vi "Initial.vi"() -> (1 "flag":i32[](array[numeric]), 2 "Output cluster":T1)   [LabVIEW 2016]
uses:
  Model Management/Global_MdlMgmt.vi
  Communication/Global communication.vi
  <vilib>/imath/engines/lvmath2/RunTimeEngine/Managers/WorkSpace/UID Generator.vi
  <vilib>/imath/engines/lvmath2/RunTimeEngine/BuiltInFunctions/size/NIMS_[I32,I32]=size(GM).vi
  <vilib>/imath/engines/lvmath2/RunTimeEngine/RangeToken/NIMS_Range_R2 - Integer.vi
  <vilib>/imath/engines/lvmath2/RunTimeEngine/IndexRead/NIMS M(S,S).vi
  <vilib>/imathl/engines/lvmath/Functions/Error Handling/Create Error.vi
  <vilib>/imath/engines/lvmath2/RunTimeEngine/CommandStatement/MC_CommandStatement_break.vi
  <vilib>/imath/engines/lvmath2/RunTimeEngine/IndexRead/NIMS M($,S).vi
  <vilib>/imath/engines/lvmath2/RunTimeEngine/BuiltInFunctions/findnz/NIMS_[3o]_findnz(GColV).vi
  <vilib>/imath/engines/lvmath2/RunTimeEngine/ErrorHandling/NIMS_Create Error From Enums.vi
  <vilib>/imath/engines/lvmath2/RunTimeEngine/BuiltInFunctions/is_empty/NIMS_is_empty(GV).vi
  <vilib>/imath/engines/lvmath2/RunTimeEngine/BuiltInFunctions/size/NIMS_[I32,I32]=size(GCol).vi
  <vilib>/imath/engines/lvmath2/RunTimeEngine/IndexRead/NIMS V(S).vi
  <vilib>/imath/engines/lvmath2/RunTimeEngine/IndexRead/NIMS M(R2,$).vi
  <vilib>/imath/engines/lvmath2/RunTimeEngine/LocalVariableDefStatement/MC_LocalVariableDefStatement_Display.vi
  <vilib>/imath/engines/lvmath2/RunTimeEngine/RunTimeType/NIMS_RunTimeType_From StrictType (excl LVString).vi
  <vilib>/imath/engines/lvmath2/RunTimeEngine/IndexReplace/NIMS M(S,S)=S.vi
  <vilib>/imath/engines/lvmath2/RunTimeEngine/IndexRead/NIMS M(S,$).vi
  <vilib>/imath/engines/lvmath2/RunTimeEngine/MatrixToken/NIMS_MatrixToken_M_RV.vi
  <vilib>/imath/engines/lvmath2/RunTimeEngine/BuiltInFunctions/zeros/NIMS_V=zeros(I32,I32).vi
  <vilib>/imath/engines/lvmath2/RunTimeSupport/NIMS_Error if Not Equal.vi
  <vilib>/imath/engines/lvmath2/RunTimeEngine/IndexReplace/NIMS V(S)=S.vi
  <vilib>/imath/engines/lvmath2/RunTimeEngine/Managers/SymbolTable/Clear UID.vi
  <vilib>/imath/engines/lvmath2/RunTimeEngine/Managers/SymbolTable/NIMS_WorkSpace.lvlib
  <vilib>/imath/engines/lvmath2/RunTimeEngine/NodeEndStatement/NIMS_NodeEndStatement_Output.vi
  <vilib>/imath/engines/lvmath2/RunTimeEngine/ErrorHandling/NIMS_Finalize Error.vi
panel:
  in  "Tnumber":dbl=8.0
  out "PVmax":dbl
  out "fixedQ":dbl
  out "fixedP":dbl
  in  "PVramp":dbl=1000.0
  in  "maxV":dbl=1.05
  in  "minV":dbl=0.95
  in  "minf":dbl=59.5
  in  "maxf":dbl=60.5
  in  "Array 2":dbl[][](array[numeric])=[[1.0, 2.0, 3.0, 0.0, 100.0, 0.0, 0.0, 0.0, 0.0, 0.0, 0.0, 0.0, 0.0, 0.0, 0.0, 0.0], [2.0, 3.0, 1.0, 0.0, 1.0, 0.0, 0.0, 0.0, 0.0, 0.0, 0.0, 0.0, 0.0, 0.0, 0.0, 0.0], [3.0, 4.0, 1.0, 1.0, 2.0, 0.0, 0.0, 0.0, 0.0, 0.0, 0.0, 0.0, 0.0, 0.0, 0.0, 0.0], [4.0, 5.0, 1.0, 0.0, 4.0, 0.0, 0.0, 0.0, 0.0, 0.0, 0.0, 0.0, 0.0, 0.0, 0.0, 0.0], [4.0, 6.0, 3.0, 0.0, 100.0, 0.0, 0.0, 0.0, 0.0, 0.0, 0.0, 1.0, 2.0, 3.0, 0.0, 100.0], [3.0, 7.0, 1.0, 0.0, 3.0, 0.0, 0.0, 0.0, 0.0, 0.0, 0.0, 2.0, 3.0, 1.0, 0.0, 1.0], [7.0, 8.0, 1.0, 0.0, 5.0, 0.0, 0.0, 0.0, 0.0, 0.0, 0.0, 3.0, 4.0, 1.0, 0.0, 2.0], [7.0, 9.0, 1.0, 0.0, 6.0, 0.0, 0.0, 0.0, 0.0, 0.0, 0.0, 4.0, 5.0, 1.0, 0.0, 4.0], [9.0, 10.0, 1.0, 0.0, 7.0, 0.0, 0.0, 0.0, 0.0, 0.0, 0.0, 4.0, 6.0, 3.0, 0.0, 100.0], [10.0, 13.0, 2.0, 0.0, 100.0, 0.0, 0.0, 0.0, 0.0, 0.0, 0.0, 3.0, 7.0, 1.0, 0.0, 3.0], [10.0, 12.0, 2.0, 0.0, 100.0, 0.0, 0.0, 0.0, 0.0, 0.0, 0.0, 7.0, 8.0, 1.0, 0.0, 5.0], [10.0, 11.0, 1.0, 0.0, 8.0, 0.0, 0.0, 0.0, 0.0, 0.0, 0.0, 7.0, 9.0, 1.0, 0.0, 6.0], [11.0, 14.0, 3.0, 0.0, 100.0, 0.0, 0.0, 0.0, 0.0, 0.0, 0.0, 9.0, 10.0, 1.0, 0.0, 7.0], [0.0, 0.0, 0.0, 0.0, 0.0, 0.0, 0.0, 0.0, 0.0, 0.0, 0.0, 10.0, 13.0, 2.0, 0.0, 100.0], [0.0, 0.0, 0.0, 0.0, 0.0, 0.0, 0.0, 0.0, 0.0, 0.0, 0.0, 10.0, 12.0, 2.0, 0.0, 100.0], [0.0, 0.0, 0.0, 0.0, 0.0, 0.0, 0.0, 0.0, 0.0, 0.0, 0.0, 10.0, 11.0, 1.0, 0.0, 8.0], [0.0, 0.0, 0.0, 0.0, 0.0, 0.0, 0.0, 0.0, 0.0, 0.0, 0.0, 11.0, 14.0, 3.0, 0.0, 100.0]]
  out "error out":errorcluster
  in  "Array":dbl[][](array[numeric])=[[1.0, 0.0, 1.0, 0.0, 0.0, 0.0, 0.0, 0.0, 0.0, 0.0, 0.0, 0.0, 0.0, 0.0, 0.0, 0.0], [0.0, 0.0, 0.0, 0.0, 0.0, 0.0, 0.0, 0.0, 0.0, 0.0, 0.0, 0.0, 0.0, 0.0, 0.0, 0.0], [0.0, 0.0, 1.0, 1.0, 0.0, 0.0, 0.0, 0.0, 0.0, 0.0, 0.0, 0.0, 0.0, 0.0, 0.0, 0.0], [0.0, 0.0, 0.0, 0.0, 0.0, 0.0, 0.0, 0.0, 0.0, 0.0, 0.0, 0.0, 0.0, 0.0, 0.0, 0.0], [0.0, 0.0, 0.0, 0.0, 0.0, 0.0, 0.0, 0.0, 0.0, 0.0, 0.0, 1.0, 2.0, 3.0, 0.0, 100.0], [0.0, 0.0, 0.0, 0.0, 0.0, 0.0, 0.0, 0.0, 0.0, 0.0, 0.0, 2.0, 3.0, 1.0, 0.0, 1.0], [0.0, 0.0, 0.0, 0.0, 0.0, 0.0, 0.0, 0.0, 0.0, 0.0, 0.0, 3.0, 4.0, 1.0, 0.0, 2.0], [0.0, 0.0, 0.0, 0.0, 0.0, 0.0, 0.0, 0.0, 0.0, 0.0, 0.0, 4.0, 5.0, 1.0, 0.0, 4.0], [0.0, 0.0, 0.0, 0.0, 0.0, 0.0, 0.0, 0.0, 0.0, 0.0, 0.0, 4.0, 6.0, 3.0, 0.0, 100.0], [0.0, 0.0, 0.0, 0.0, 0.0, 0.0, 0.0, 0.0, 0.0, 0.0, 0.0, 3.0, 7.0, 1.0, 0.0, 3.0], [0.0, 0.0, 0.0, 0.0, 0.0, 0.0, 0.0, 0.0, 0.0, 0.0, 0.0, 7.0, 8.0, 1.0, 0.0, 5.0], [0.0, 0.0, 0.0, 0.0, 0.0, 0.0, 0.0, 0.0, 0.0, 0.0, 0.0, 7.0, 9.0, 1.0, 0.0, 6.0], [0.0, 0.0, 0.0, 0.0, 0.0, 0.0, 0.0, 0.0, 0.0, 0.0, 0.0, 9.0, 10.0, 1.0, 0.0, 7.0], [0.0, 0.0, 0.0, 0.0, 0.0, 0.0, 0.0, 0.0, 0.0, 0.0, 0.0, 10.0, 13.0, 2.0, 0.0, 100.0], [0.0, 0.0, 0.0, 0.0, 0.0, 0.0, 0.0, 0.0, 0.0, 0.0, 0.0, 10.0, 12.0, 2.0, 0.0, 100.0], [0.0, 0.0, 0.0, 0.0, 0.0, 0.0, 0.0, 0.0, 0.0, 0.0, 0.0, 10.0, 11.0, 1.0, 0.0, 8.0], [0.0, 0.0, 0.0, 0.0, 0.0, 0.0, 0.0, 0.0, 0.0, 0.0, 0.0, 11.0, 14.0, 3.0, 0.0, 100.0]]
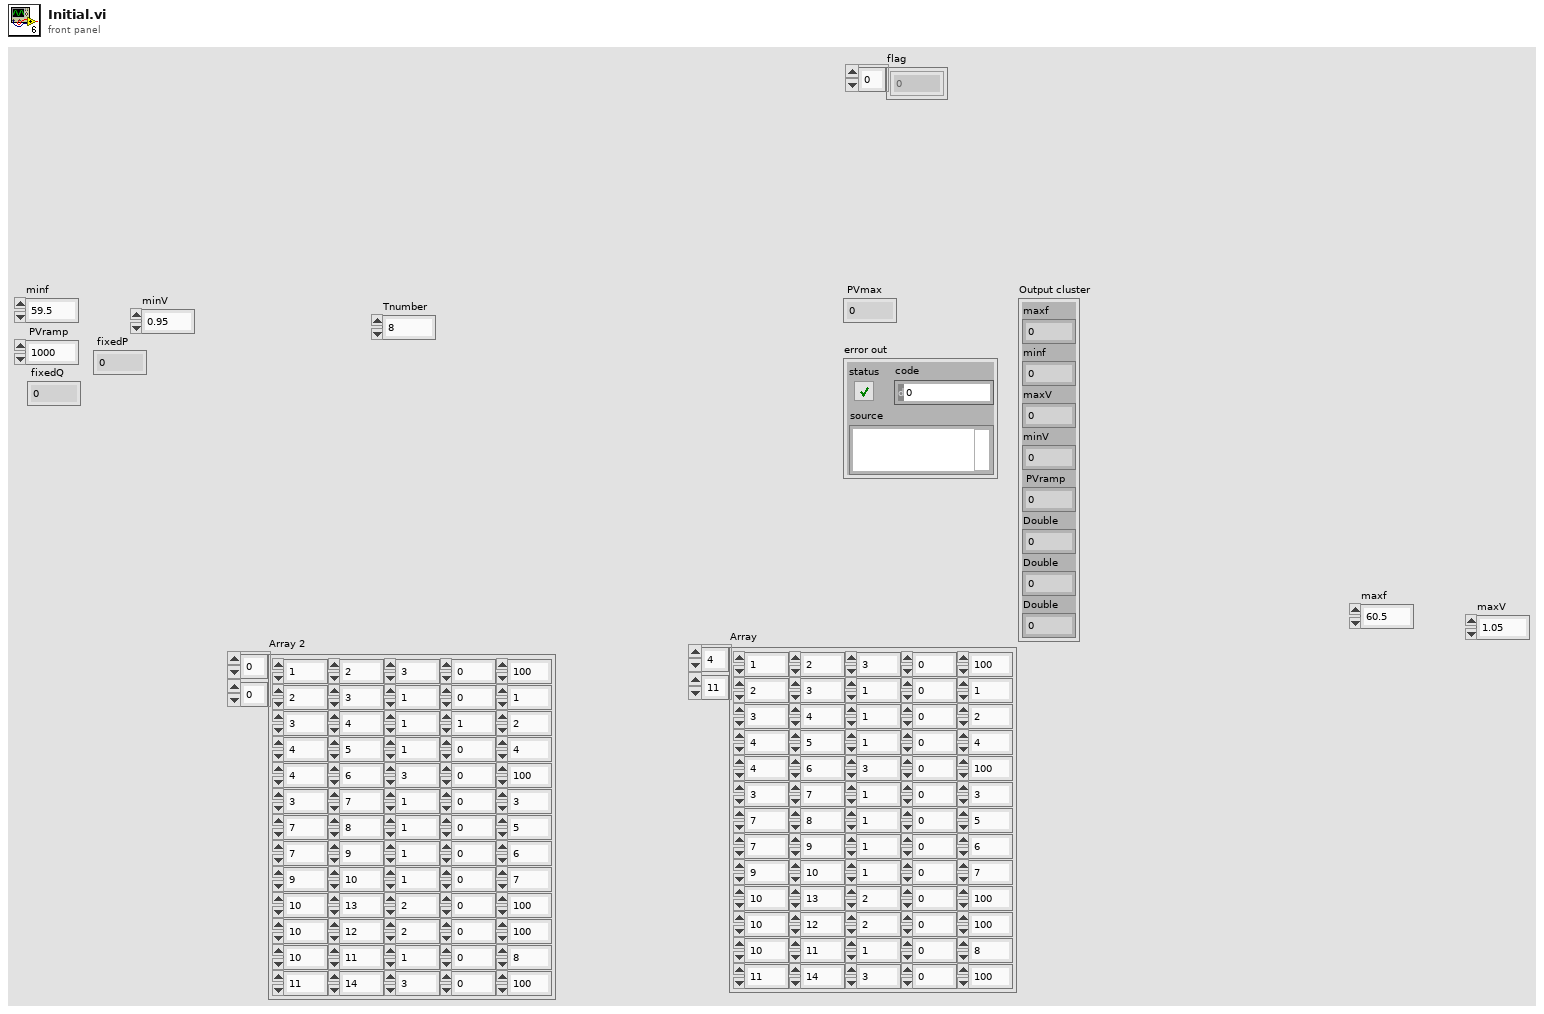
[diagram p1: front panel]
types:
  T1 = cluster{"maxf":dbl, "minf":dbl, "maxV":dbl, "minV":dbl, " PVramp":dbl, "Double":dbl, "Double":dbl, "Double":dbl}
  T2 = cluster{"BESS max Freq":dbl, "BESS min Freq":dbl, "BESS max Vol":dbl, "BESS min Vol":dbl, " PVramp":dbl, "Double":dbl, "fixP":dbl, "fixQ":dbl}
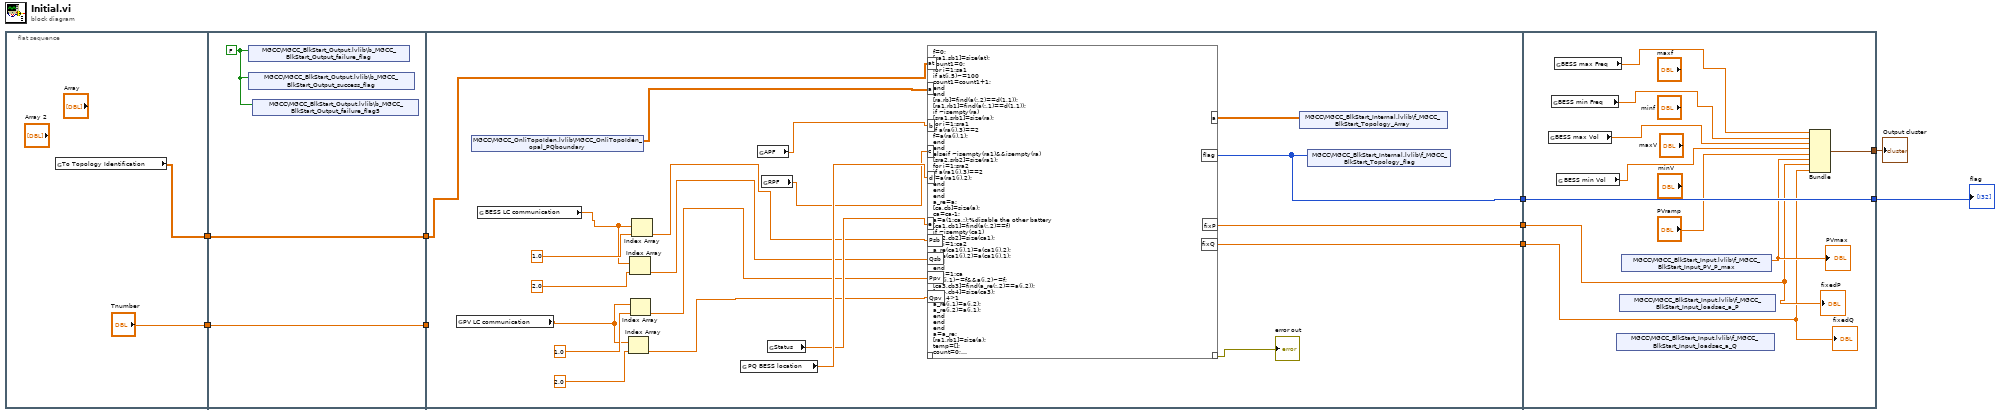
[diagram p0: block diagram]
diagram:
  n1 = flat-sequence {
    tunnel: [w10] -> w5
    tunnel: ["Tnumber"] -> w3
    tunnel: [w14] -> w6
    tunnel: w5 -> [w14]
    tunnel: [w13] -> w4
    tunnel: w3 -> [w13]
    tunnel: [w33] -> w9
    tunnel: w6 -> [w17]
    tunnel: w4 -> [_]
    tunnel: [w28] -> w2
    tunnel: [w27] -> w1
    tunnel: [w1798] -> w8
    tunnel: w9 -> [w1798]
    tunnel: [w1795] -> w7
    tunnel: w2 -> [w1790]
    tunnel: w1 -> [w1789]
    frame #0 {
      n2 = global read "Global_MdlMgmt.vi" "To Topology Identification"() -> (w10:dbl[][])
    }
    frame #1 {
      w12 = FALSE
      n3 = shared-variable "MGCC\\MGCC_BlkStart_Output.lvlib\\b_MGCC_BlkStart_Output_failure_flag"(w12) -> ()  [unwired: 1 in, 1 out]
      n4 = shared-variable "MGCC\\MGCC_BlkStart_Output.lvlib\\b_MGCC_BlkStart_Output_success_flag"(w12) -> ()  [unwired: 1 in, 1 out]
      n5 = shared-variable "MGCC\\MGCC_BlkStart_Output.lvlib\\b_MGCC_BlkStart_Output_failure_flag5"(w12) -> ()  [unwired: 1 in, 1 out]
    }
    frame #2 {
      n6 = global read "Global communication.vi" "PV LC communication"() -> (w15:dbl[])
      n7 = shared-variable "MGCC\\MGCC_OnliTopoIden.lvlib\\MGCC_OnliTopoIden_opal_PQboundary"() -> (w18:dbl[][])  [unwired: 1 in, 1 out]
      n8 = global read "Global communication.vi" "BESS LC communication"() -> (w16:dbl[])
      n9 = Index Array(array=w15, index=2.0) -> (element=w19:dbl)
      n10 = Index Array(array=w16, index=2.0) -> (element=w21:dbl)
      n11 = Index Array(array=w15, index=1.0) -> (element=w20:dbl)
      n12 = Index Array(array=w16, index=1.0) -> (element=w22:dbl)
      n13 = global read "Global_MdlMgmt.vi" "PQ BESS location"() -> (w32:dbl[])
      n14 = global read "Global communication.vi" "APF"() -> (w30:dbl[])
      n15 = global read "Global communication.vi" "RPF"() -> (w29:dbl[])
      n16 = global read "Global communication.vi" "Status"() -> (w31:dbl[])
      n17 = mathscript code="f=0;\n[sa1,sb1]=size(at);\ncount1=0;\nfor i=1:sa1\nif at(i,5)~=100\ncount1=count1+1;\nend\nend\n[ra,rb]=find(a(:,2)==d(1,1));\n[ra1,rb1]=find(a(:,1)==d(1,1));\nif ~isempty(ra)\n[sra1,srb1]=size(ra);\nfor i=1:sra1\nif a(ra(i),3)==2\nf=a(ra(i),1);\nend\nend\nelseif ~isempty(ra1)&&isempty(ra)\n[sra2,srb2]=size(ra1);\nfor i=1:sra2\nif a(ra1(i),3)==2\nf=a(ra1(i),2);\nend\nend\nend\na_re=a;\n[ca,cb]=size(a);\nca=ca-1;\na=a(1:ca,:);%disable the other battery\n[ca1,cb1]=find(a(:,2)==f)\nif ~isempty(ca1)\n[ca2,cb2]=size(ca1);\nfor i=1:ca2\na_re(ca1(i),1)=a(ca1(i),2);\na_re(ca1(i),2)=a(ca1(i),1);\nend\nend\nfor i=1:ca\nif a(i,1)~=f&&a(i,2)~=f;\n[ca3,cb3]=find(a_re(:,2)==a(i,2));\n[ca4,cb4]=size(ca3);\nif ca4>1\na_re(i,1)=a(i,2);\na_re(i,2)=a(i,1);\nend\nend\nend\na=a_re;\n[ra1,rb1]=size(a);\ntemp=[];\ncount=0;\nfor i=1:ra1\nif a(i,3)~=2&&a(i,3)~=4\ncount=count+1;\ntemp=[temp;a(i,:)];\nend\nend\na=temp;\nflag=zeros(count1,1);\nfor i=1:count\nif a(i,3)==1\nflag(a(i,5))=1;\nend\nend\nfixP=0;\nfixQ=0;\n[ra7,rb7]=size(temp);\n[fa1,fb1]=find(a(:,1)==f)\n[ra2,rb2]=size(fa1);\nif ~isempty(ra2)\nfor i=1:ra2\nif a(fa1(i),3)==2\nfixP=fixP+Psb;\nfixQ=fixQ+Qsb;\nelseif a(fa1(i),3)==4\nfixP=fixP+Ppv;\nfixQ=fixQ+Qpv;\nelse\n[fa2,fb2]=find(temp(:,2)==a(fa1(i),2));\n[ra7,rb7]=size(fa2);\nif ra7==1\nfor j=1:ra7\nfixP=fixP-b(fa2(j));\nfixQ=fixQ-c(fa2(j));\nend\nend\nend\nend\nend"("a"=w18, "b"=w30, "c"=w29, "d"=w32, "e"=w31, "Psb"=w22, "Qsb"=w21, "Ppv"=w20, "Qpv"=w19, "at"=w17) -> ("??"=→"error out":errorcluster, "a"=w35:dbl[][], "flag"=w33:i32[], "fixP"=w28:dbl, "fixQ"=w27:dbl)  [unwired: 1 in]
      n18 = shared-variable "MGCC\\MGCC_BlkStart_Internal.lvlib\\f_MGCC_BlkStart_Topology_Array"(w35) -> ()  [unwired: 1 in, 1 out]
      n19 = shared-variable "MGCC\\MGCC_BlkStart_Internal.lvlib\\f_MGCC_BlkStart_Topology_flag"(w33) -> ()  [unwired: 1 in, 1 out]
    }
    frame #3 {
      n20 = global read "Global_MdlMgmt.vi" "BESS max Vol"() -> (w1792:dbl)
      n21 = global read "Global_MdlMgmt.vi" "BESS min Freq"() -> (w1793:dbl)
      n22 = global read "Global_MdlMgmt.vi" "BESS max Freq"() -> (w1794:dbl)
      n23 = global read "Global_MdlMgmt.vi" "BESS min Vol"() -> (w1791:dbl)
      n24 = shared-variable "MGCC\\MGCC_BlkStart_Input.lvlib\\f_MGCC_BlkStart_Input_loadsec_a_Q"() -> ()  [unwired: 1 in, 2 out]
      n25 = shared-variable "MGCC\\MGCC_BlkStart_Input.lvlib\\f_MGCC_BlkStart_Input_loadsec_a_P"() -> ()  [unwired: 1 in, 2 out]
      n26 = shared-variable "MGCC\\MGCC_BlkStart_Input.lvlib\\f_MGCC_BlkStart_Input_PV_P_max"() -> (w1796:dbl)  [unwired: 1 in, 1 out]
      "PVmax" <- w1796
      n27 = Bundle("BESS max Freq"=w1794, "BESS min Freq"=w1793, "BESS max Vol"=w1792, "BESS min Vol"=w1791, "PVramp"="PVramp", "Double"=w1796, "fixP"=w1790, "fixQ"=w1789) -> (w1795:T2)  [unwired: 1 in]
      "fixedP" <- w1790
      "fixedQ" <- w1789
    }
  }
  "flag" <- w8
  "Output cluster" <- w7
